vi "Open CSM_Tool_Launcher.vi"() -> ()   [LabVIEW 2014, in "csm_tool_menu.lvlib"]
uses:
  csm_tool_menu.lvlib
panel:
  out "appended path":path
  in  "error in (no error)":errorcluster
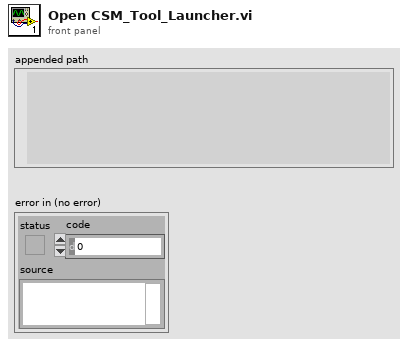
[diagram p1: front panel]
types:
  T1 = enum32{"Invalid", "Standard", "Closed", "Hidden", "Minimized", "Maximized"}
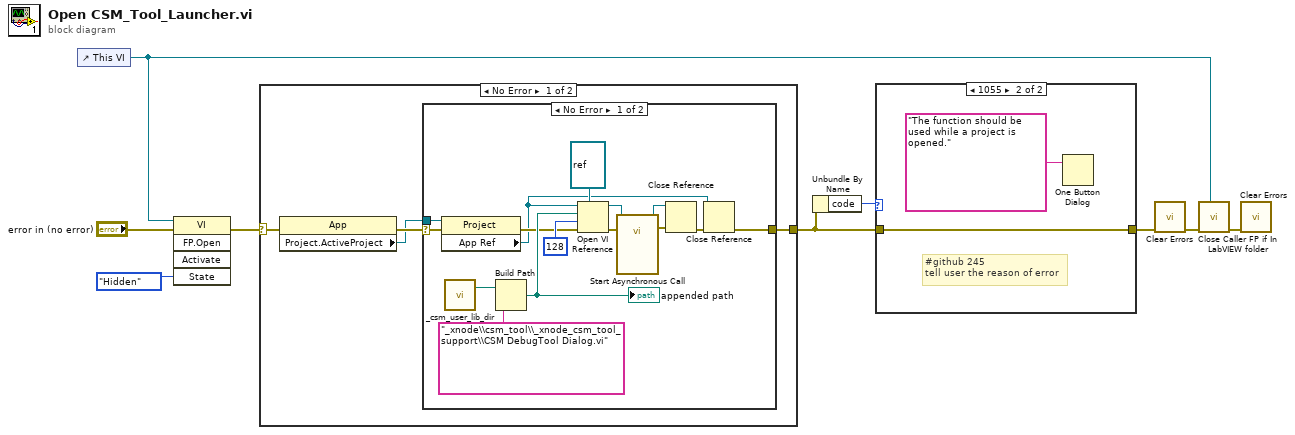
[diagram p0: block diagram]
diagram:
  n1 = control-ref of="This VI"() -> (w4:refnum<vi>)
  n2 = invoke class="VI" method="FP.Open"(reference=w4, error in="error in (no error)", "State"=T1."Hidden") -> (error out=w5:errorcluster)  [unwired: 2 in, 4 out]
  n3 = case shown="No Error" w5 {
    selector: w5 -> [w13 w30]
    tunnel: [w12 w30] -> w2
    frame No Error {
      n4 = property class="App"(error in=w13) -> (error out=w11:errorcluster, "Project.ActiveProject"=w10:refnum<vi>)  [unwired: 1 in, 1 out]
      n5 = case shown="No Error" w11 {
        selector: w11 -> [w19 w29]
        tunnel: [w15 w29] -> w12
        tunnel: w10 -> [w18 _]
        frame No Error {
          n6 = property class="Project"(reference=w18, error in=w19) -> (error out=w17:errorcluster, "App Ref"=w14:refnum<vi>)  [unwired: 1 out]
          n7 = call "_csm_user_lib_dir.vi"() -> ("csm_user.lib_dir"=w22:path)  [unwired: 2 in, 1 out]
          n8 = Build Path(base path=w22, name or relative path="_xnode\\csm_tool\\_xnode_csm_tool_support\\CSM DebugTool Dialog.vi") -> (appended path=w23:path)
          "appended path" <- w23
          n9 = Open VI Reference(type specifier VI Refnum (for type only)=refnum<vi> refnum, application reference (local)=w14, vi path=w23, options=128, error in (no error)=w17) -> (vi reference=w25:refnum<vi>, error out=w24:errorcluster)  [unwired: 1 in]
          n10 = call-by-ref "Start Asynchronous Call"(reference=w25, error in=w24) -> (reference out=w27:refnum<vi>, error out=w26:errorcluster)  [unwired: 12 in]
          n11 = Close Reference(reference=w27, error in (no error)=w26) -> (error out=w16:errorcluster)
          n12 = Close Reference(reference=w14, error in (no error)=w16) -> (error out=w15:errorcluster)
        }
        frame Error {
        }
      }
    }
    frame Error {
    }
  }
  n13 = Unbundle By Name(w2) -> ("code"=w1:i32)
  n14 = case shown="1055" w1 {
    tunnel: w2 -> [w31 w33]
    tunnel: [w31 w33] -> w3
    frame 0, Default {
    }
    frame 1055 {
      # "#github 245\ntell user the reason of error"
      n15 = One Button Dialog(message="The function should be used while a project is opened.") -> ()  [unwired: 1 in, 1 out]
    }
  }
  n16 = call <vilib>:"Clear Errors.vi"("error in (no error)"=w3) -> ("error out"=w8:errorcluster)  [unwired: 6 in]
  n17 = call "Close Caller FP if In LabVIEW folder.vi"("VI Ref"=w4, "error in (no error)"=w8) -> ("error out"=w9:errorcluster)  [unwired: 9 in]
  n18 = call <vilib>:"Clear Errors.vi"("error in (no error)"=w9) -> ()  [unwired: 6 in, 1 out]
